vi "fetch-frame-data-from-dbc.vi"(8 "error in (no error)":errorcluster, 11 "frame.tag":string) -> (0 "error out":errorcluster, 3 "frame":T1={"Comment"="", "Extended Identifier?"=FALSE, "Transmit Time"=0.0, "Timing Type"=1, "Payload Length"=8, "Identifier"=1, "Frame name"="frame1"} {"Timing Type" items=["Cyclic Data", "Event Data", "Cyclic Remote", "Event Remote"]; "Identifier" format="%010x"})   [LabVIEW 2015]
doc: "Use this template to build a VI to use as a subVI."
uses:
  controls/dbc-frame.ctl
  <vilib>/xnet/xnet.llb/XNET String To IO Name (Frame).vi
  <resource>/objmgr/xnet.rc
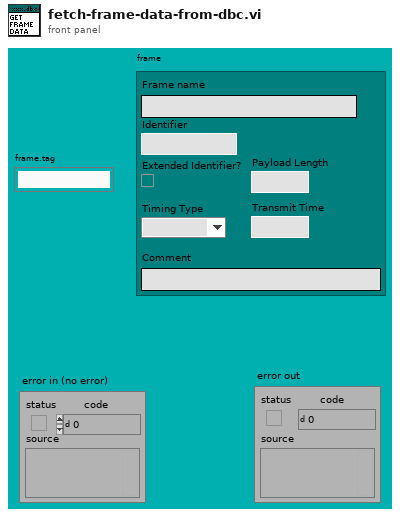
[diagram p1: front panel]
types:
  T1 = typedef "dbc-frame.ctl" = cluster{"Comment":string, "Extended Identifier?":bool, "Transmit Time":dbl, "Timing Type":u32, "Payload Length":u32, "Identifier":u32, "Frame name":string}
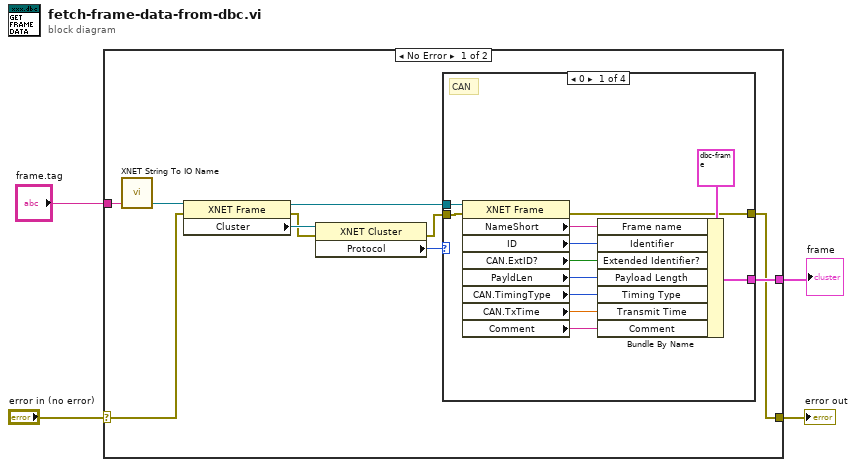
[diagram p0: block diagram]
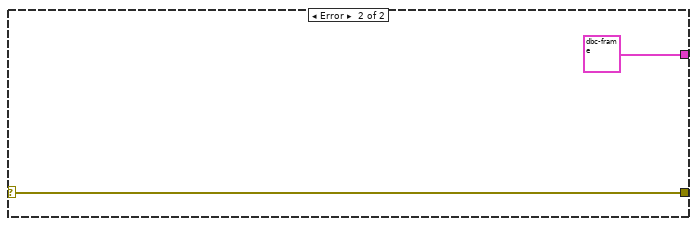
[diagram p5: hidden frame]
diagram:
  n1 = case shown="No Error" "error in (no error)" {
    selector: "error in (no error)" -> [w10 w31]
    tunnel: [w9 w31] -> w3
    tunnel: "frame.tag" -> [w14 _]
    tunnel: [w12 T1 {"Comment"="frame not found", "Extended Identifier?"=FALSE, "Transmit Time"=0.0, "Timing Type"=1, "Payload Length"=8, "Identifier"=1, "Frame name"="frame1"} ("CAN Cluster")] -> w1
    frame No Error {
      n2 = call-poly <vilib>:"XNET String To IO Name.vi"("string"=w14) -> ("XNET Frame"=w13:refnum<k21>)  [unwired: 4 out]
      n3 = property class="XNET Frame"(reference=w13, error in=w10) -> (reference out=w11:refnum<k21>, error out=w6:errorcluster, "Cluster"=w8:refnum<k21>)
      n4 = property class="XNET Cluster"(reference=w8, error in=w6) -> (error out=w5:errorcluster, "Protocol"=w7:u32)  [unwired: 1 out]
      n5 = case shown="0" w7 {
        tunnel: [w25 _ _ _] -> w12
        tunnel: w11 -> [w24 _ _ _]
        tunnel: w5 -> [w23 w27 w28 w29]
        tunnel: [w22 w27 w28 w29] -> w9
        frame 0 {
          # "CAN"
          n6 = property class="XNET Frame"(reference=w24, error in=w23) -> (error out=w22:errorcluster, "NameShort"=w21:string, "ID"=w20:u32, "CAN.ExtID?"=w19:bool, "PayldLen"=w18:u32, "CAN.TimingType"=w17:u32, "CAN.TxTime"=w16:dbl, "Comment"=w15:string)  [unwired: 1 out]
          n7 = Bundle By Name(cluster=T1 {"Comment"="", "Extended Identifier?"=FALSE, "Transmit Time"=0.0, "Timing Type"=1, "Payload Length"=8, "Identifier"=1, "Frame name"="frame1"} ("CAN Cluster"), "Frame name"=w21, "Identifier"=w20, "Extended Identifier?"=w19, "Payload Length"=w18, "Timing Type"=w17, "Transmit Time"=w16, "Comment"=w15) -> (w25:T1)
        }
        frame 1 {
          # "flexray"
        }
        frame 2 {
          # "LIN"
        }
        frame Default {
          # "undefined"
        }
      }
    }
    frame Error {
    }
  }
  "error out" <- w3
  "frame" <- w1
